vi "Write Single Bit.vi"(8 "error in (no error)":errorcluster, 9 "ON/OFF":bool, 10 "Address":u16=65535 format="%.0x", 11 "Port Selection Info":T1={"Port Name"="", "Amplifier Num"=1, "Baud Rate"=38400, "Char Formation"=enum."0"} {"Baud Rate" items=["38400"=38400, "19200"=19200, "9600"=9600, "115200"=0]; "Amplifier Num" max=31}) -> (0 "error out":errorcluster, 3 "Port Selection Info Out":T1={"Port Name"="", "Amplifier Num"=1, "Baud Rate"=38400, "Char Formation"=enum."0"} {"Baud Rate" items=["38400"=38400, "19200"=19200, "9600"=9600, "115200"=0]; "Amplifier Num" max=31})   [LabVIEW 2014, in "ALPHA5 RS485.lvlib"]
uses:
  ALPHA5 RS485.lvlib
  typedefs/Port Selection Info.ctl
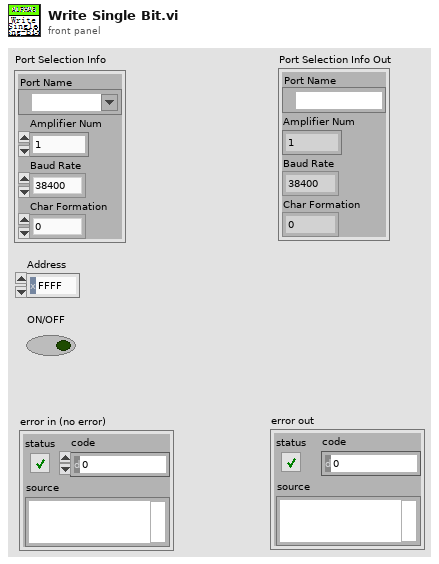
[diagram p1: front panel]
types:
  T1 = typedef "ALPHA5 RS485.lvlib/Port Selection Info.ctl" = cluster{"Port Name":refnum<visa-resource-name>, "Amplifier Num":u8, "Baud Rate":u32, "Char Formation":enum16{"0", "1", "2", "3", "4", "5"}}
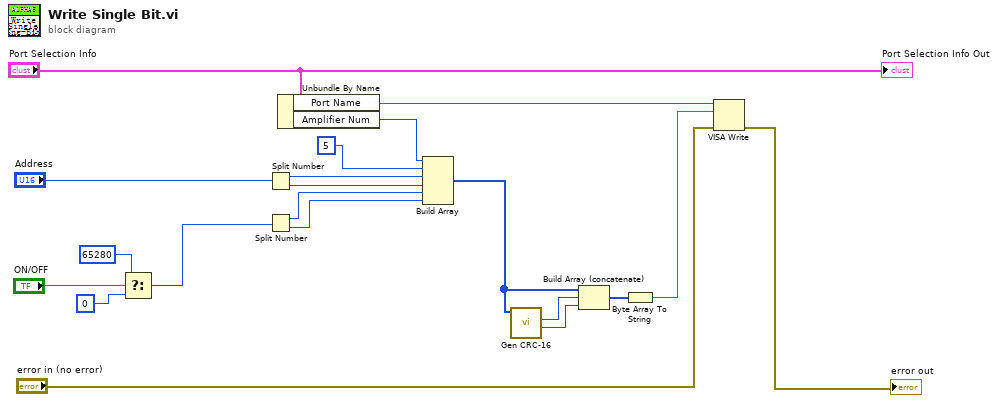
[diagram p0: block diagram]
diagram:
  n1 = Select(t=u16 65280, s="ON/OFF", f=u16 0) -> (s? t:f=w1:u16)
  n2 = Split Number(x="Address") -> (hi(x)=w14:u8, lo(x)=w13:u8)
  n3 = Split Number(x=w1) -> (hi(x)=w12:u8, lo(x)=w11:u8)
  n4 = Unbundle By Name("Port Selection Info") -> ("Port Name"=w6:refnum<visa-resource-name>, "Amplifier Num"=w15:u8)
  n5 = Build Array(w15, u8 5 ("FC"), w14, w13, w12, w11) -> (w7:u8[])
  n6 = call "Gen CRC-16.vi"("Data In"=w7) -> ("CRC-16-H"=w9:u8, "CRC-16-L"=w10:u8)  [unwired: 7 in, 2 out]
  n7 = Build Array (concatenate)(w7, w10, w9) -> (w8:u8[])
  n8 = Byte Array To String(unsigned byte array=w8) -> (string=w5:string)
  n9 = VISA Write(VISA resource name=w6, write buffer=w5, error in (no error)="error in (no error)") -> (error out=→"error out":errorcluster)  [unwired: 2 out]
  "Port Selection Info Out" <- "Port Selection Info"
